vi "ASG8x00.vi"() -> ()   [LabVIEW 2020]
uses:
  ASG8X00_Win32.dll
  Labview Library/Libraries/ASG8100CY/ASG8X00_x64.dll
panel:
  out "value":u32[](array[numeric])
  in  "IN2":dbl
  out "start 3":bool
  out "length":dbl
  out "segment":dbl
  out "channel":dbl
  out "错误码内容":string
  out "错误码长度":dbl
  out "错误类型值":dbl
  in  "ASG使能按钮":bool
  in  "ASG使能":dbl
  in  "ASG长高电平开关":bool
  in  "长高电平":dbl
  in  "停止播放":bool
  in  "播放按钮":bool
  in  "下载COUNT":bool
  in  "下载ASG":bool
  in  "COUNT文件 *.count":path
  in  "ASG文件  *.pulse":path
  in  "循环次数":dbl
  in  "配置模式":bool
  in  "IN1":dbl
  out "连接状态":bool
  in  "断开按钮":bool
  in  "连接按钮":bool
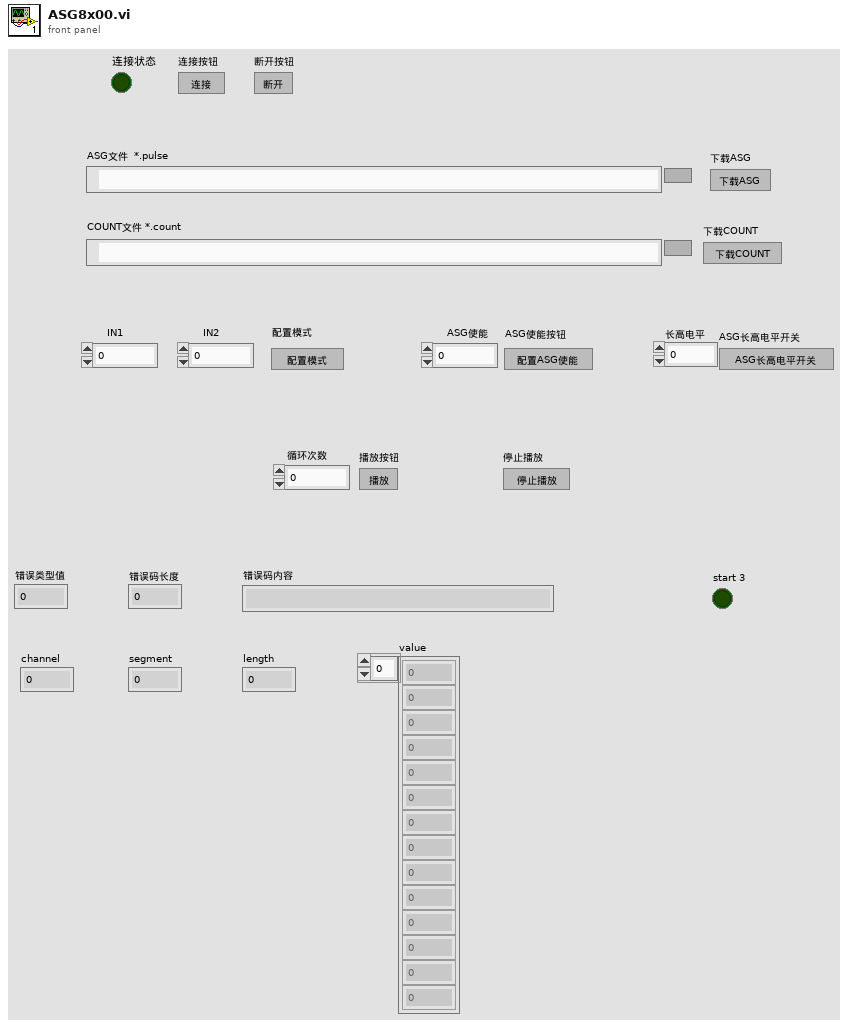
[diagram p1: front panel]
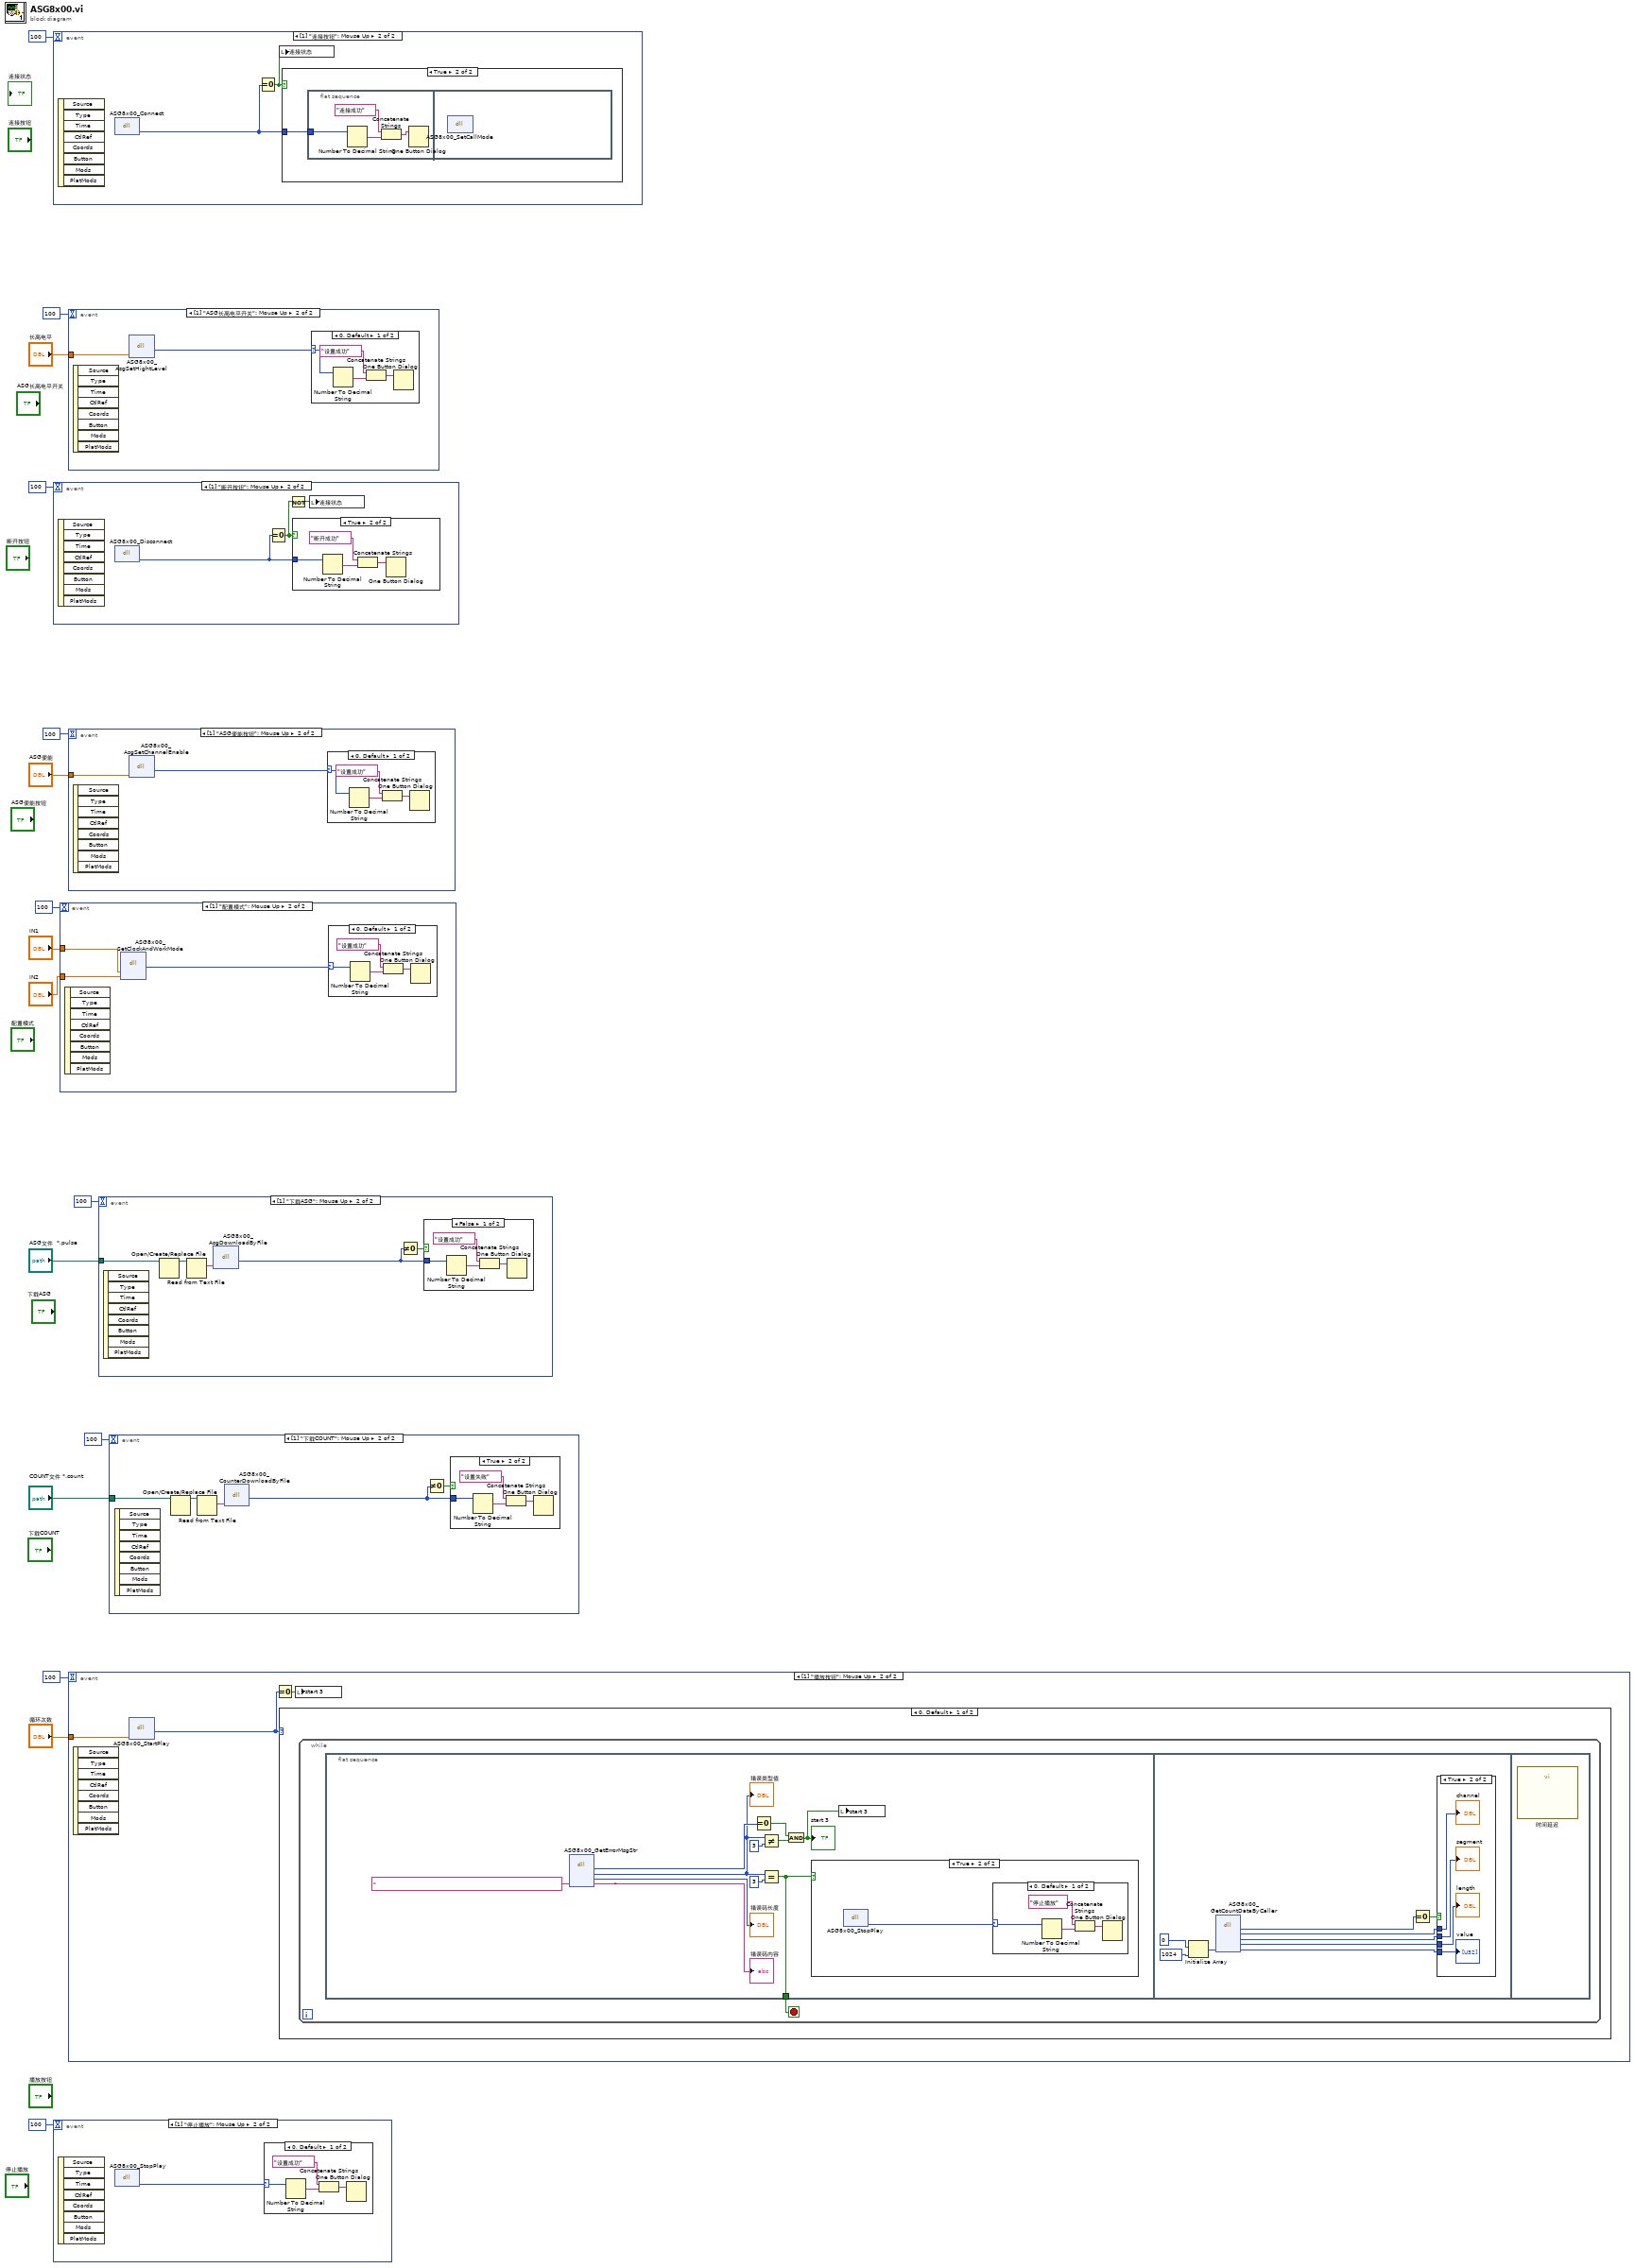
[diagram p0: block diagram]
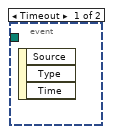
[diagram p2: hidden frame]
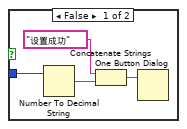
[diagram p3: hidden frame]
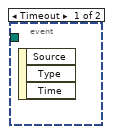
[diagram p4: hidden frame]
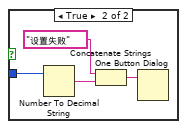
[diagram p5: hidden frame]
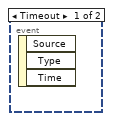
[diagram p6: hidden frame]
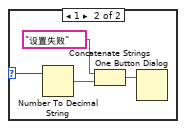
[diagram p7: hidden frame]
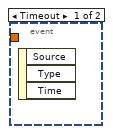
[diagram p8: hidden frame]
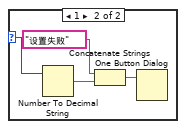
[diagram p9: hidden frame]
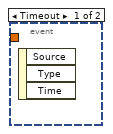
[diagram p10: hidden frame]
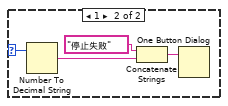
[diagram p12: hidden frame]
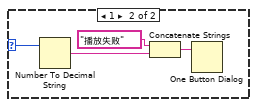
[diagram p14: hidden frame]
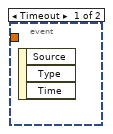
[diagram p15: hidden frame]
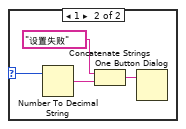
[diagram p16: hidden frame]
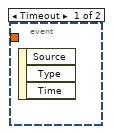
[diagram p17: hidden frame]
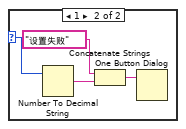
[diagram p18: hidden frame]
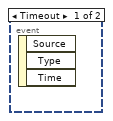
[diagram p19: hidden frame]
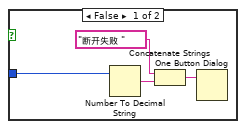
[diagram p20: hidden frame]
diagram:
  n1 = event shown="[1] \"连接按钮\": Mouse Up" {
    selector: _ -> [_ _]
    dyn-events: _ -> [_ _]
    timeout: 100 -> [_ _]
    event Timeout {
      n2 = event-data() -> ()  [unwired: 1 in, 3 out]
    }
    event "连接按钮": Mouse Up {
      n3 = event-data() -> ()  [unwired: 1 in, 8 out]
      n4 = dll-call lib="F:/Labview Library/Libraries/ASG8100CY/ASG8X00_x64.dll" fn="ASG8x00_Connect"() -> ("返回类型"=w18:i32)  [unwired: 3 in, 2 out]
      n5 = Equal To 0?(x=w18) -> (x = 0?=w17:bool)
      n6 = local write "连接状态"(w17) -> ()
      n7 = case shown="True" w17 {
        tunnel: w18 -> [w19 w23]
        frame False {
          n8 = Number To Decimal String(number=w19) -> (decimal integer string=w20:string)  [unwired: 1 in]
          n9 = Concatenate Strings("连接设备失败 ", w20) -> (w21:string)
          n10 = One Button Dialog(message=w21) -> ()  [unwired: 1 in, 1 out]
        }
        frame True {
          n11 = flat-sequence {
            tunnel: w23 -> [w24]
            frame #0 {
              n12 = Number To Decimal String ("数值至十进制数字符串转换")(number=w24) -> (decimal integer string=w26:string)  [unwired: 1 in]
              n13 = Concatenate Strings("连接成功", w26) -> (w27:string)
              n14 = One Button Dialog(message=w27) -> ()  [unwired: 1 in, 1 out]
            }
            frame #1 {
              n15 = dll-call lib="F:/Labview Library/Libraries/ASG8100CY/ASG8X00_x64.dll" fn="ASG8x00_SetCallMode"() -> ()  [unwired: 4 in, 2 out]
            }
          }
        }
      }
    }
  }
  n16 = event shown="[1] \"断开按钮\": Mouse Up" {
    selector: _ -> [_ _]
    dyn-events: _ -> [_ _]
    timeout: 100 -> [_ _]
    event Timeout {
      n17 = event-data() -> ()  [unwired: 1 in, 3 out]
    }
    event "断开按钮": Mouse Up {
      n18 = event-data() -> ()  [unwired: 1 in, 8 out]
      n19 = dll-call lib="F:/Labview Library/Libraries/ASG8100CY/ASG8X00_x64.dll" fn="ASG8x00_Disconnect"() -> ("返回类型"=w30:i32)  [unwired: 3 in, 2 out]
      n20 = Equal To 0?(x=w30) -> (x = 0?=w28:bool)
      n21 = Not(x=w28) -> (.not. x?=w29:bool)
      n22 = case shown="True" w28 {
        tunnel: w30 -> [w31 w35]
        frame False {
          n23 = Number To Decimal String(number=w31) -> (decimal integer string=w32:string)  [unwired: 1 in]
          n24 = Concatenate Strings("断开失败 ", w32) -> (w33:string)
          n25 = One Button Dialog(message=w33) -> ()  [unwired: 1 in, 1 out]
        }
        frame True {
          n26 = Number To Decimal String ("数值至十进制数字符串转换")(number=w35) -> (decimal integer string=w37:string)  [unwired: 1 in]
          n27 = Concatenate Strings("断开成功", w37) -> (w38:string)
          n28 = One Button Dialog(message=w38) -> ()  [unwired: 1 in, 1 out]
        }
      }
      n29 = local write "连接状态"(w29) -> ()
    }
  }
  n30 = event shown="[1] \"停止播放\": Mouse Up" {
    selector: _ -> [_ _]
    dyn-events: _ -> [_ _]
    timeout: 100 -> [_ _]
    event Timeout {
      n31 = event-data() -> ()  [unwired: 1 in, 3 out]
    }
    event "停止播放": Mouse Up {
      n32 = event-data() -> ()  [unwired: 1 in, 8 out]
      n33 = dll-call lib="C:/Users/Administrator/Desktop/ASG8x00/ASG8100/ASG8x00_labview/ASG8X00_Win32.dll" fn="ASG8x00_StopPlay"() -> ("返回类型"=w39:i32)  [unwired: 3 in, 2 out]
      n34 = case shown="0, Default" w39 {
        selector: w39 -> [w40 w44]
        frame 0, Default {
          n35 = Number To Decimal String ("数值至十进制数字符串转换")(number=w40) -> (decimal integer string=w42:string)  [unwired: 1 in]
          n36 = Concatenate Strings("设置成功", w42) -> (w41:string)
          n37 = One Button Dialog(message=w41) -> ()  [unwired: 1 in, 1 out]
        }
        frame 1 {
          n38 = Number To Decimal String ("数值至十进制数字符串转换")(number=w44) -> (decimal integer string=w46:string)  [unwired: 1 in]
          n39 = Concatenate Strings("设置失败", w46) -> (w45:string)
          n40 = One Button Dialog(message=w45) -> ()  [unwired: 1 in, 1 out]
        }
      }
    }
  }
  n41 = event shown="[1] \"配置模式\": Mouse Up" {
    selector: _ -> [_ _]
    dyn-events: _ -> [_ _]
    timeout: 100 -> [_ _]
    tunnel: "IN1" -> [_ w50]
    tunnel: "IN2" -> [_ w48]
    event Timeout {
      n42 = event-data() -> ()  [unwired: 1 in, 3 out]
    }
    event "配置模式": Mouse Up {
      n43 = event-data() -> ()  [unwired: 1 in, 8 out]
      n44 = dll-call lib="C:/Users/Administrator/Desktop/ASG8x00/ASG8100/ASG8x00_labview/ASG8X00_Win32.dll" fn="ASG8x00_SetClockAndWorkMode"("IN1"=w50, "IN2"=w48) -> ("返回类型"=w49:i32)  [unwired: 5 in, 2 out]
      n45 = case shown="0, Default" w49 {
        selector: w49 -> [w51 w55]
        frame 0, Default {
          n46 = Number To Decimal String ("数值至十进制数字符串转换")(number=w51) -> (decimal integer string=w53:string)  [unwired: 1 in]
          n47 = Concatenate Strings("设置成功", w53) -> (w52:string)
          n48 = One Button Dialog(message=w52) -> ()  [unwired: 1 in, 1 out]
        }
        frame 1 {
          n49 = Number To Decimal String ("数值至十进制数字符串转换")(number=w55) -> (decimal integer string=w57:string)  [unwired: 1 in]
          n50 = Concatenate Strings("设置失败", w57) -> (w56:string)
          n51 = One Button Dialog(message=w56) -> ()  [unwired: 1 in, 1 out]
        }
      }
    }
  }
  n52 = event shown="[1] \"ASG长高电平开关\": Mouse Up" {
    selector: _ -> [_ _]
    dyn-events: _ -> [_ _]
    timeout: 100 -> [_ _]
    tunnel: "长高电平" -> [_ w60]
    event Timeout {
      n53 = event-data() -> ()  [unwired: 1 in, 3 out]
    }
    event "ASG长高电平开关": Mouse Up {
      n54 = event-data() -> ()  [unwired: 1 in, 8 out]
      n55 = dll-call lib="C:/Users/Administrator/Desktop/ASG8x00/ASG8100/ASG8x00_labview/ASG8X00_Win32.dll" fn="ASG8x00_AsgSetHightLevel"("参数1"=w60) -> ("返回类型"=w59:i32)  [unwired: 4 in, 2 out]
      n56 = case shown="0, Default" w59 {
        selector: w59 -> [w61 w65]
        frame 0, Default {
          n57 = Number To Decimal String ("数值至十进制数字符串转换")(number=w61) -> (decimal integer string=w63:string)  [unwired: 1 in]
          n58 = Concatenate Strings("设置成功", w63) -> (w62:string)
          n59 = One Button Dialog(message=w62) -> ()  [unwired: 1 in, 1 out]
        }
        frame 1 {
          n60 = Number To Decimal String ("数值至十进制数字符串转换")(number=w65) -> (decimal integer string=w67:string)  [unwired: 1 in]
          n61 = Concatenate Strings("设置失败", w67) -> (w66:string)
          n62 = One Button Dialog(message=w66) -> ()  [unwired: 1 in, 1 out]
        }
      }
    }
  }
  n63 = event shown="[1] \"ASG使能按钮\": Mouse Up" {
    selector: _ -> [_ _]
    dyn-events: _ -> [_ _]
    timeout: 100 -> [_ _]
    tunnel: "ASG使能" -> [_ w70]
    event Timeout {
      n64 = event-data() -> ()  [unwired: 1 in, 3 out]
    }
    event "ASG使能按钮": Mouse Up {
      n65 = event-data() -> ()  [unwired: 1 in, 8 out]
      n66 = dll-call lib="C:/Users/Administrator/Desktop/ASG8x00/ASG8100/ASG8x00_labview/ASG8X00_Win32.dll" fn="ASG8x00_AsgSetChannelEnable"("参数1"=w70) -> ("返回类型"=w69:i32)  [unwired: 4 in, 2 out]
      n67 = case shown="0, Default" w69 {
        selector: w69 -> [w71 w75]
        frame 0, Default {
          n68 = Number To Decimal String ("数值至十进制数字符串转换")(number=w71) -> (decimal integer string=w73:string)  [unwired: 1 in]
          n69 = Concatenate Strings("设置成功", w73) -> (w72:string)
          n70 = One Button Dialog(message=w72) -> ()  [unwired: 1 in, 1 out]
        }
        frame 1 {
          n71 = Number To Decimal String ("数值至十进制数字符串转换")(number=w75) -> (decimal integer string=w77:string)  [unwired: 1 in]
          n72 = Concatenate Strings("设置失败", w77) -> (w76:string)
          n73 = One Button Dialog(message=w76) -> ()  [unwired: 1 in, 1 out]
        }
      }
    }
  }
  n74 = event shown="[1] \"播放按钮\": Mouse Up" {
    selector: _ -> [_ _]
    dyn-events: _ -> [_ _]
    timeout: 100 -> [_ _]
    tunnel: "循环次数" -> [_ w81]
    event Timeout {
      n75 = event-data() -> ()  [unwired: 1 in, 3 out]
    }
    event "播放按钮": Mouse Up {
      n76 = event-data() -> ()  [unwired: 1 in, 8 out]
      n77 = dll-call lib="C:/Users/Administrator/Desktop/ASG8x00/ASG8100/ASG8x00_labview/ASG8X00_Win32.dll" fn="ASG8x00_StartPlay"("参数1"=w81) -> ("返回类型"=w80:i32)  [unwired: 4 in, 2 out]
      n78 = Equal To 0?(x=w80) -> (x = 0?=w79:bool)
      n79 = case shown="0, Default" w80 {
        selector: w80 -> [_ w116]
        frame 0, Default {
          n80 = while {
            stop <- w82 stop-if-true
            n81 = flat-sequence {
              tunnel: [w83] -> w82
              frame #0 {
                n82 = dll-call lib="C:/Users/Administrator/Desktop/ASG8x00/ASG8100/ASG8x00_labview/ASG8X00_Win32.dll" fn="ASG8x00_GetErrorMsgStr"("str_value"="                                                                                                                              ") -> ("返回类型"=w92:i32, "type"=w84:i32, "length"=→"错误码长度":i32, "str_value"=→"错误码内容":string)  [unwired: 5 in, 2 out]
                "错误类型值" <- w84
                n83 = Equal To 0?(x=w92) -> (x = 0?=w90:bool)
                n84 = Not Equal?(x=w84, y=3) -> (x != y?=w86:bool)
                n85 = Equal?(x=w84, y=3) -> (x = y?=w83:bool)
                n86 = And(x=w90, y=w86) -> (x .and. y?=w91:bool)
                "start 3" <- w91
                n87 = case shown="True" w83 {
                  frame False {
                  }
                  frame True {
                    n88 = dll-call lib="C:/Users/Administrator/Desktop/ASG8x00/ASG8100/ASG8x00_labview/ASG8X00_Win32.dll" fn="ASG8x00_StopPlay"() -> ("返回类型"=w94:i32)  [unwired: 3 in, 2 out]
                    n89 = case shown="0, Default" w94 {
                      selector: w94 -> [w95 w99]
                      frame 0, Default {
                        n90 = Number To Decimal String ("数值至十进制数字符串转换")(number=w95) -> (decimal integer string=w97:string)  [unwired: 1 in]
                        n91 = Concatenate Strings("停止播放", w97) -> (w96:string)
                        n92 = One Button Dialog(message=w96) -> ()  [unwired: 1 in, 1 out]
                      }
                      frame 1 {
                        n93 = Number To Decimal String ("数值至十进制数字符串转换")(number=w99) -> (decimal integer string=w101:string)  [unwired: 1 in]
                        n94 = Concatenate Strings("停止失败", w101) -> (w100:string)
                        n95 = One Button Dialog(message=w100) -> ()  [unwired: 1 in, 1 out]
                      }
                    }
                  }
                }
                n96 = local write "start 3"(w91) -> ()
              }
              frame #1 {
                n97 = Initialize Array(0, 1024) -> (w111:i32[])
                n98 = dll-call lib="C:/Users/Administrator/Desktop/ASG8x00/ASG8100/ASG8x00_labview/ASG8X00_Win32.dll" fn="ASG8x00_GetCountDataByCaller"("value"=w111) -> ("返回类型"=w106:i32, "channel"=w105:i32, "segment"=w103:i32, "length"=w104:i32, "value"=w108:u32[])  [unwired: 6 in, 2 out]
                n99 = Equal To 0?(x=w106) -> (x = 0?=w107:bool)
                n100 = case shown="True" w107 {
                  tunnel: w108 -> [_ w113]
                  tunnel: w105 -> [_ w115]
                  tunnel: w104 -> [_ w112]
                  tunnel: w103 -> [_ w114]
                  frame False {
                  }
                  frame True {
                    "value" <- w113
                    "segment" <- w114
                    "length" <- w112
                    "channel" <- w115
                  }
                }
              }
              frame #2 {
                n101 = call "时间延迟"() -> ()  [unwired: 11 in, 1 out]
              }
            }
          }
        }
        frame 1 {
          n102 = Number To Decimal String ("数值至十进制数字符串转换")(number=w116) -> (decimal integer string=w118:string)  [unwired: 1 in]
          n103 = Concatenate Strings("播放失败", w118) -> (w117:string)
          n104 = One Button Dialog(message=w117) -> ()  [unwired: 1 in, 1 out]
        }
      }
      n105 = local write "start 3"(w79) -> ()
    }
  }
  n106 = event shown="[1] \"下载ASG\": Mouse Up" {
    selector: _ -> [_ _]
    dyn-events: _ -> [_ _]
    timeout: 100 -> [_ _]
    tunnel: "ASG文件  *.pulse" -> [_ w124]
    event Timeout {
      n107 = event-data() -> ()  [unwired: 1 in, 3 out]
    }
    event "下载ASG": Mouse Up {
      n108 = event-data() -> ()  [unwired: 1 in, 8 out]
      n109 = Open/Create/Replace File(file path (use dialog)=w124) -> (refnum out=w121:refnum<file>)  [unwired: 5 in, 2 out]
      n110 = Read from Text File(file (use dialog)=w121) -> (text=w120:string)  [unwired: 3 in, 3 out]
      n111 = dll-call lib="F:/Labview Library/Libraries/ASG8100CY/ASG8X00_x64.dll" fn="ASG8x00_AsgDownloadByFile"("参数1"=w120) -> ("返回类型"=w122:i32)  [unwired: 4 in, 2 out]
      n112 = Not Equal To 0?(x=w122) -> (x != 0?=w123:bool)
      n113 = case shown="False" w123 {
        tunnel: w122 -> [w125 w129]
        frame False {
          n114 = Number To Decimal String ("数值至十进制数字符串转换")(number=w125) -> (decimal integer string=w127:string)  [unwired: 1 in]
          n115 = Concatenate Strings("设置成功", w127) -> (w126:string)
          n116 = One Button Dialog(message=w126) -> ()  [unwired: 1 in, 1 out]
        }
        frame True {
          n117 = Number To Decimal String ("数值至十进制数字符串转换")(number=w129) -> (decimal integer string=w131:string)  [unwired: 1 in]
          n118 = Concatenate Strings("设置失败", w131) -> (w130:string)
          n119 = One Button Dialog(message=w130) -> ()  [unwired: 1 in, 1 out]
        }
      }
    }
  }
  n120 = event shown="[1] \"下载COUNT\": Mouse Up" {
    selector: _ -> [_ _]
    dyn-events: _ -> [_ _]
    timeout: 100 -> [_ _]
    tunnel: "COUNT文件 *.count" -> [_ w137]
    event Timeout {
      n121 = event-data() -> ()  [unwired: 1 in, 3 out]
    }
    event "下载COUNT": Mouse Up {
      n122 = event-data() -> ()  [unwired: 1 in, 8 out]
      n123 = Open/Create/Replace File(file path (use dialog)=w137) -> (refnum out=w136:refnum<file>)  [unwired: 5 in, 2 out]
      n124 = Read from Text File(file (use dialog)=w136) -> (text=w135:string)  [unwired: 3 in, 3 out]
      n125 = dll-call lib="C:/Users/Administrator/Desktop/ASG8x00/ASG8100/ASG8x00_labview/ASG8X00_Win32.dll" fn="ASG8x00_CounterDownloadByFile"("参数1"=w135) -> ("返回类型"=w133:i32)  [unwired: 4 in, 2 out]
      n126 = Not Equal To 0?(x=w133) -> (x != 0?=w134:bool)
      n127 = case shown="True" w134 {
        tunnel: w133 -> [w138 w142]
        frame False {
          n128 = Number To Decimal String ("数值至十进制数字符串转换")(number=w138) -> (decimal integer string=w140:string)  [unwired: 1 in]
          n129 = Concatenate Strings("设置成功", w140) -> (w139:string)
          n130 = One Button Dialog(message=w139) -> ()  [unwired: 1 in, 1 out]
        }
        frame True {
          n131 = Number To Decimal String ("数值至十进制数字符串转换")(number=w142) -> (decimal integer string=w144:string)  [unwired: 1 in]
          n132 = Concatenate Strings("设置失败", w144) -> (w143:string)
          n133 = One Button Dialog(message=w143) -> ()  [unwired: 1 in, 1 out]
        }
      }
    }
  }
